vi "terminate.vi"(8 "error in (no error)":errorcluster, 11 "DL090324Microscope in":refnum<class "InstrumentDL090324.lvclass">) -> (0 "error out":errorcluster, 3 "DL090324Microscope out":refnum<class "InstrumentDL090324.lvclass">)   [LabVIEW 2010, in "InstrumentDL090324.lvclass"]
uses:
  InstrumentDL090324.lvclass
  InstrumentDL090324.lvclass/InstrumentDL090324.ctl
  Detector/GenericDetector/GenericDetector/GenericDetector.lvclass
  LightSource/GenericLightSource/GenericLightSource/GenericLightSource.lvclass
  GenericInstrument/GenericInstrument/GenericInstrument.lvclass
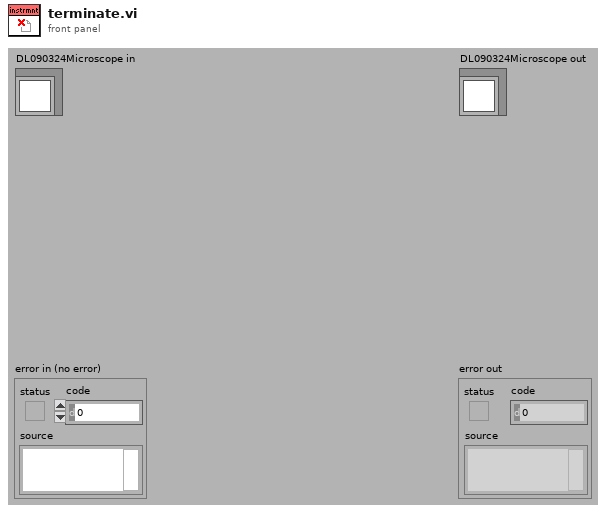
[diagram p1: front panel]
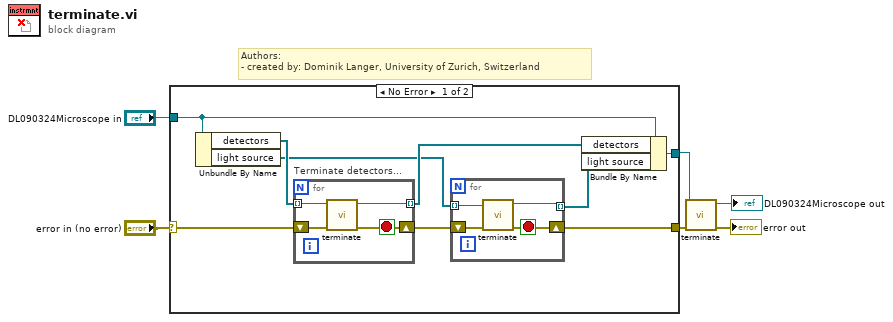
[diagram p0: block diagram]
diagram:
  # "Authors: \n- created by: Dominik Langer, University of Zurich, Switzerland"
  n1 = case shown="No Error" "error in (no error)" {
    selector: "error in (no error)" -> [w14 w25]
    tunnel: [w7 w25] -> w4
    tunnel: [w12 w24] -> w1
    tunnel: "DL090324Microscope in" -> [w13 w24]
    frame No Error {
      n2 = Unbundle By Name(w13) -> ("detectors"=w15:refnum<class "GenericDetector.lvclass">[], "light source"=w10:refnum<class "GenericLightSource.lvclass">[])
      n3 = for "Terminate detectors..." {
        shift-right: [w20] -> w8
        shift-left: w14 -> [w23]
        tunnel: w15 -> [w22] mode=indexing
        tunnel: [w21] -> w11 mode=indexing
        stop <- w20 stop-if-true
        n4 = call-dynamic "terminate.vi"("error in (no error)"=w23, "GenericPlugin in"=w22) -> ("error out"=w20:errorcluster, "GenericPlugin out"=w21:refnum<class "GenericDetector.lvclass">)  [unwired: 8 out]
      }
      n5 = for {
        tunnel: w10 -> [w18] mode=indexing
        tunnel: [w17] -> w9 mode=indexing
        shift-right: [w16] -> w7
        shift-left: w8 -> [w19]
        stop <- w16 stop-if-true
        n6 = call-dynamic "terminate.vi"("error in (no error)"=w19, "GenericPlugin in"=w18) -> ("error out"=w16:errorcluster, "GenericPlugin out"=w17:refnum<class "GenericLightSource.lvclass">)  [unwired: 8 out]
      }
      n7 = Bundle By Name(cluster=w13, "detectors"=w11, "light source"=w9) -> (w12:refnum<class "InstrumentDL090324.lvclass">)
    }
    frame Error {
    }
  }
  n8 = call-parent "terminate.vi"("error in (no error)"=w4, "GenericPlugin in"=w1) -> ("error out"=→"error out":errorcluster, "GenericPlugin out"=→"DL090324Microscope out":refnum<class "InstrumentDL090324.lvclass">)  [unwired: 8 out]
